vi "Benchmark Convert String Type - Create Single Type Block Conversions.vi"(9 "dst data type":T1, 10 "src data type":T1, 11 "channel count":i32) -> (3 "conversions":T2[](array[typedef]) {"converted descriptor"."buffer offset" format="%d bytes"; "unconverted descriptor"."buffer offset" format="%d bytes"})   [LabVIEW 2017]
uses:
  Classes/Buffer Converter/Type Conversion.ctl
  Classes/Buffer Converter/Channel Descriptor.ctl
  DSF Configuration API/Public/Controls/DSF Data Type.ctl
  DSF Core.lvlib
  Classes/Buffer/Buffer.lvclass
  Classes/Buffer Converter/Buffer Converter.lvclass
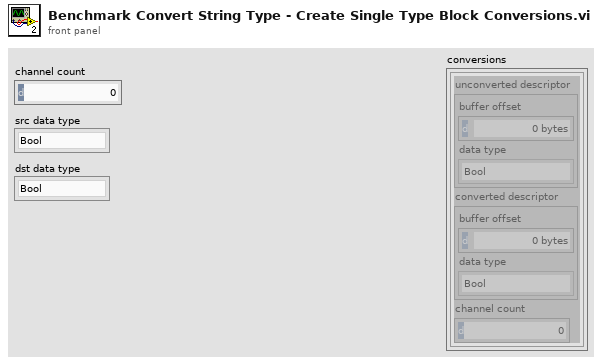
[diagram p1: front panel]
types:
  T1 = typedef "DSF Core.lvlib/DSF Data Type.ctl" = enum8{"Bool", "SGL", "DBL", "I8", "I16", "I32", "I64", "U8", "U16", "U32", "U64"}
  T2 = typedef "DSF Core.lvlib/Buffer Converter.lvclass/Type Conversion.ctl" = cluster{"unconverted descriptor":T3, "converted descriptor":T3, "channel count":u64}
  T3 = typedef "DSF Core.lvlib/Buffer.lvclass/Channel Descriptor.ctl" = cluster{"buffer offset":u64, "data type":T1}
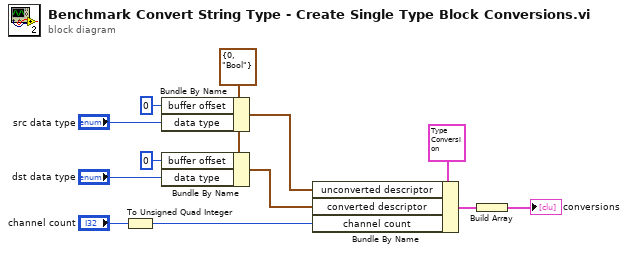
[diagram p0: block diagram]
diagram:
  w3 = T3 {"buffer offset"=0, "data type"=enum."Bool"} ("unconverted descriptor")
  n1 = To Unsigned Quad Integer(1:"channel count") -> (0:w8:u64)
  n2 = Bundle By Name(cluster=w3, "buffer offset"=u64 0, "data type"="src data type") -> (w12:T3)
  n3 = Bundle By Name(cluster=w3, "buffer offset"=u64 0, "data type"="dst data type") -> (w11:T3)
  n4 = Bundle By Name(cluster=T2 {"unconverted descriptor"={"buffer offset"=0, "data type"=enum."Bool"}, "converted descriptor"={"buffer offset"=0, "data type"=enum."Bool"}, "channel count"=0} ("conversion"), "unconverted descriptor"=w12, "converted descriptor"=w11, "channel count"=w8) -> (w2:T2)
  n5 = Build Array(w2) -> (→"conversions":T2[])
